vi "Calculate IM Freq.vi"(1 "Low-side?":bool, 2 "F2 (Carrier 2)":dbl, 3 "F1 (Carrier 1)":dbl, 4 "BaseImOrder":i32) -> (0 "IM Frequency":dbl)   [LabVIEW 2011]
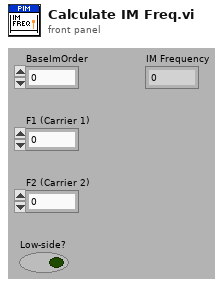
[diagram p1: front panel]
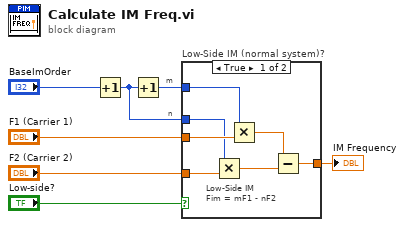
[diagram p0: block diagram]
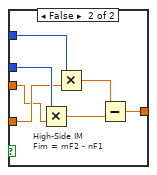
[diagram p2: hidden frame]
diagram:
  # "n"
  # "m"
  n1 = Increment(x="BaseImOrder") -> (x+1=w6:i32)
  n2 = Increment(x=w6) -> (x+1=w5:i32)
  n3 = case "Low-Side IM (normal system)?" shown="True" "Low-side?" {
    tunnel: "F1 (Carrier 1)" -> [w12 w17]
    tunnel: w5 -> [w11 w21]
    tunnel: [w10 w20] -> w2
    tunnel: "F2 (Carrier 2)" -> [w9 w18]
    tunnel: w6 -> [w8 w19]
    frame True {
      # "Low-Side IM\nFim = mF1 - nF2"
      n4 = Multiply(x=w8, y=w9) -> (x*y=w13:dbl)
      n5 = Multiply(x=w11, y=w12) -> (x*y=w14:dbl)
      n6 = Subtract(x=w14, y=w13) -> (x-y=w10:dbl)
    }
    frame False {
      # "High-Side IM\nFim = mF2 - nF1"
      n7 = Multiply(x=w19, y=w17) -> (x*y=w15:dbl)
      n8 = Multiply(x=w21, y=w18) -> (x*y=w16:dbl)
      n9 = Subtract(x=w16, y=w15) -> (x-y=w20:dbl)
    }
  }
  "IM Frequency" <- w2
